vi "CRYAPI TAB PANEL RESIZE.vi"(10 "Pane Origin":T4, 11 "Pane Bound":T3) -> (2 "SubPanel Container Bound":T2, 3 "SubPanel Position":T1)   [LabVIEW 2013]
uses:
  <vilib>/Utility/miscctls.llb/LVPointTypeDef.ctl
  <vilib>/Utility/miscctls.llb/LVRectTypeDef.ctl
  <vilib>/Utility/miscctls.llb/LVBoundsTypeDef.ctl
  <vilib>/Utility/miscctls.llb/LVPositionTypeDef.ctl
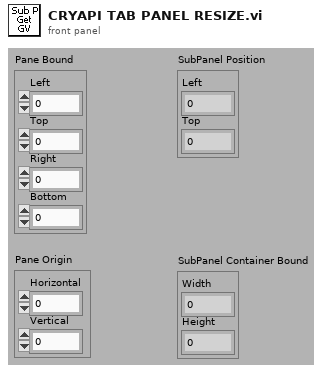
[diagram p1: front panel]
types:
  T1 = typedef "LVPositionTypeDef.ctl" = cluster{"Left":i32, "Top":i32}
  T2 = typedef "LVBoundsTypeDef.ctl" = cluster{"Width":u32, "Height":u32}
  T3 = typedef "LVRectTypeDef.ctl" = cluster{"Left":i16, "Top":i16, "Right":i16, "Bottom":i16}
  T4 = typedef "LVPointTypeDef.ctl" = cluster{"Horizontal":i16, "Vertical":i16}
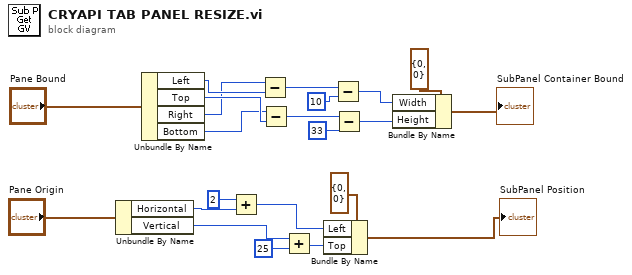
[diagram p0: block diagram]
diagram:
  n1 = Unbundle By Name("Pane Origin") -> ("Horizontal"=w15:i16, "Vertical"=w18:i16)
  n2 = Unbundle By Name("Pane Bound") -> ("Left"=w6:i16, "Top"=w8:i16, "Right"=w5:i16, "Bottom"=w7:i16)
  n3 = Add(x=i16 2, y=w15) -> (x+y=w16:i16)
  n4 = Subtract(x=w5, y=w6) -> (x-y=w11:i16)
  n5 = Subtract(x=w7, y=w8) -> (x-y=w12:i16)
  n6 = Add(x=w18, y=i16 25) -> (x+y=w19:i16)
  n7 = Bundle By Name(cluster=T1 {"Left"=0, "Top"=0} ("Position"), "Left"=w16, "Top"=w19) -> (→"SubPanel Position":T1)
  n8 = Subtract(x=w11, y=i16 10) -> (x-y=w22:i16)
  n9 = Subtract(x=w12, y=i16 33) -> (x-y=w21:i16)
  n10 = Bundle By Name(cluster=T2 {"Width"=0, "Height"=0} ("Container Bounds"), "Width"=w22, "Height"=w21) -> (→"SubPanel Container Bound":T2)
